vi "InterpolateStage1_fastPID.vi"(8 "valid in":bool, 11 "Data in":fxp<+/-,16,14>[](array[numeric])=[0.0, 0.0]) -> (0 "valid out":bool, 3 "Data out":fxp<+/-,16,14>[](array[numeric]))   [LabVIEW 2013]
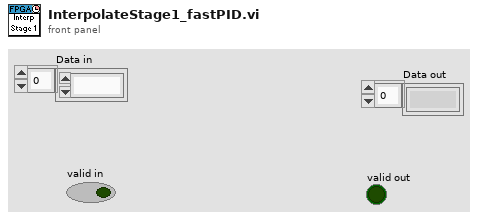
[diagram p1: front panel]
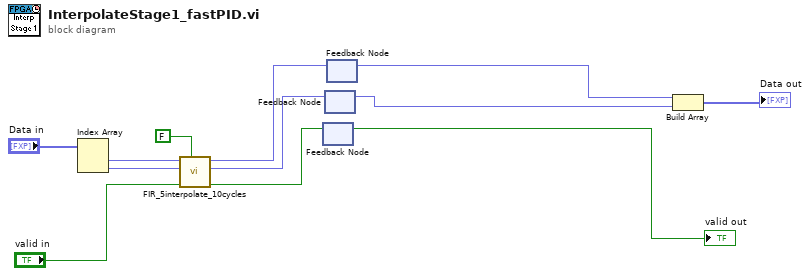
[diagram p0: block diagram]
diagram:
  n1 = Index Array(array="Data in") -> (element #1=w11:fxp<+/-,16,14>, element #2=w10:fxp<+/-,16,14>)  [unwired: 2 in]
  n2 = call "FIR_5interpolate_10cycles.vi"("reset"=FALSE, "valid in"="valid in", "Q in"=w10, "I in"=w11) -> ("valid out"=w7:bool, "Q out"=w4:fxp<+/-,16,14>, "I out"=w5:fxp<+/-,16,14>)  [unwired: 4 in, 1 out]
  n3 = feedback #1() -> (→"valid out":bool)  [unwired: 1 in]
  n4 = feedback-in #1(w7) -> ()
  n5 = feedback-in #2(w4) -> ()
  n6 = feedback #2() -> (w2:fxp<+/-,16,14>)  [unwired: 1 in]
  n7 = feedback #3() -> (w3:fxp<+/-,16,14>)  [unwired: 1 in]
  n8 = feedback-in #3(w5) -> ()
  n9 = Build Array(w3, w2) -> (→"Data out":fxp<+/-,16,14>[])
